vi "Overlay Results (Circle).vi"(5 "Setup":T2, 7 "ROI Descriptor":T1 {"Contours"."Type" items=["No Selection", "Point", "Line", "Rectangle", "Oval", "Polygon", "Free", "Annulus", "Unused2", "Unused3", "Broken Line", "Free Hand Line", "Rotated Rectangle"]}, 8 "Search Lines":T3(array[cluster]) {"?"."Y" format="%.2f"; "?"."X" format="%.2f"; "?"."Y" format="%.2f"; "?"."X" format="%.2f"}, 9 "All Edges Found":cluster{"X":sgl, "Y":sgl}[](array[cluster])=[{"X"=27.450102, "Y"=144.0}, {"X"=70.80146, "Y"=144.0}, {"X"=114.11963, "Y"=144.0}, {"X"=158.60345, "Y"=144.0}, {"X"=202.3678, "Y"=144.0}, {"X"=246.04292, "Y"=144.0}, {"X"=291.42203, "Y"=144.0}, {"X"=336.54822, "Y"=144.0}, {"X"=379.2348, "Y"=144.0}, {"X"=425.02194, "Y"=144.0}, {"X"=467.72144, "Y"=144.0}, {"X"=26.88918, "Y"=210.0}, {"X"=70.6191, "Y"=210.0}, {"X"=115.31038, "Y"=210.0}, {"X"=159.03351, "Y"=210.0}, {"X"=202.2118, "Y"=210.0}, {"X"=247.37573, "Y"=210.0}, {"X"=292.001, "Y"=210.0}, {"X"=336.55954, "Y"=210.0}, {"X"=379.72208, "Y"=210.0}, {"X"=424.86005, "Y"=210.0}, {"X"=468.8485, "Y"=210.0}, {"X"=26.897532, "Y"=309.0}, {"X"=70.88008, "Y"=309.0}, {"X"=114.93419, "Y"=309.0}, {"X"=159.13483, "Y"=309.0}, {"X"=203.12064, "Y"=309.0}, {"X"=247.9202, "Y"=309.0}, {"X"=291.07425, "Y"=309.0}, {"X"=335.25354, "Y"=309.0}, {"X"=378.88284, "Y"=309.0}, {"X"=424.06085, "Y"=309.0}, {"X"=469.80658, "Y"=309.0}] {"Y" format="%.2f"; "X" format="%.2f"}, 10 "Circle":T4 {"Radius" format="%.2f"; "Center"."Y" format="%.2f"; "Center"."X" format="%.2f"}, 11 "Image In":T5) -> (3 "Image Out":T5)   [LabVIEW 2020]
uses:
  IMAQ Image.ctl
panel:
  in  "Result Color":u32(colorbox)=16711680
  in  "Edge Locations Color":u32(colorbox)=16776960
  in  "Search Lines Color":u32(colorbox)=26367
  in  "Search Area Color":u32(colorbox)=65280
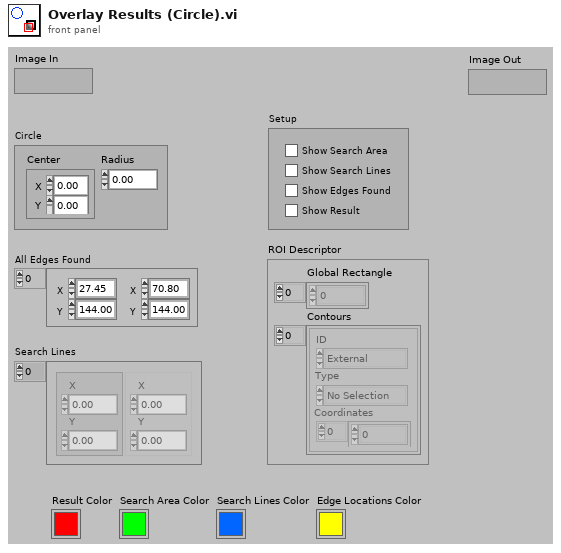
[diagram p1: front panel]
types:
  T1 = cluster{"Global Rectangle":i32[], "Contours":cluster{"ID":enum32{"External", "Internal"}, "Type":u32, "Coordinates":i32[]}[]}
  T2 = cluster{"Show Search Area":bool, "Show Search Lines":bool, "Show Edges Found":bool, "Show Result":bool}
  T3 = cluster{cluster{"X":sgl, "Y":sgl}, cluster{"X":sgl, "Y":sgl}}[]
  T4 = cluster{"Center":cluster{"X":sgl, "Y":sgl}, "Radius":dbl}
  T5 = typedef "IMAQ Image.ctl" = refnum<image>
  T6 = cluster{"[0]":sgl, "[1]":sgl, "[2]":sgl, "[3]":sgl}
  T7 = cluster{"[0]":dbl, "[1]":dbl, "[2]":dbl, "[3]":dbl}
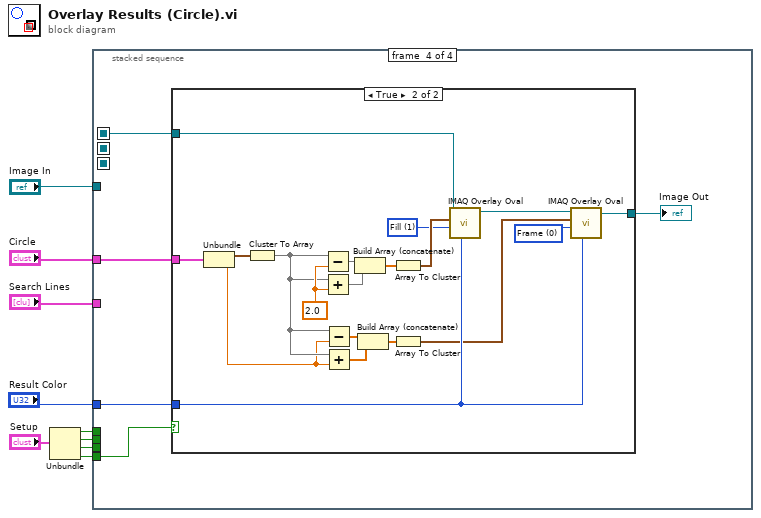
[diagram p0: block diagram]
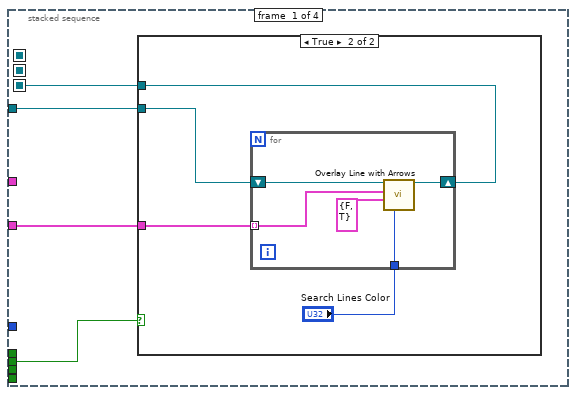
[diagram p2: hidden frame]
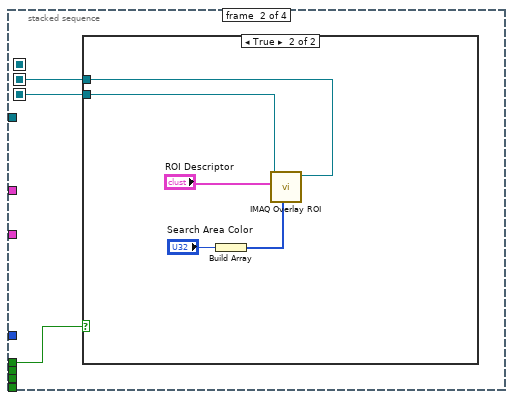
[diagram p4: hidden frame]
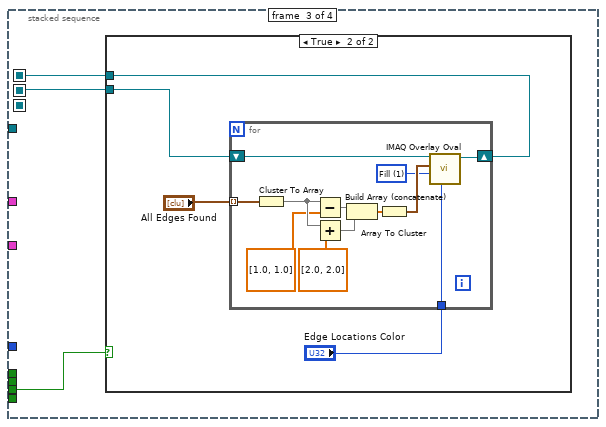
[diagram p6: hidden frame]
diagram:
  n1 = Unbundle("Setup") -> ("Show Search Area"=w3:bool, "Show Search Lines"=w4:bool, "Show Edges Found"=w2:bool, "Show Result"=w1:bool)
  n2 = stacked-sequence {
    seq-local: [_ _ w35 _] -> [_ _ _ w57]
    seq-local: [w12 _ _ _] -> [_ w25 _ _]
    seq-local: [_ w26 _ _] -> [_ _ w34 _]
    tunnel: "Image In" -> [w13 _ _ _]
    tunnel: "Search Lines" -> [w11 _ _ _]
    tunnel: "Result Color" -> [_ _ _ w56]
    tunnel: "Circle" -> [_ _ _ w55]
    tunnel: w4 -> [w10 _ _ _]
    tunnel: w3 -> [_ w24 _ _]
    tunnel: w2 -> [_ _ w33 _]
    tunnel: w1 -> [_ _ _ w54]
    frame #0 {
      n3 = case shown="True" w10 {
        tunnel: w13 -> [w14 w18]
        tunnel: [w14 w16] -> w12
        tunnel: w11 -> [_ w15]
        frame False {
        }
        frame True {
          n4 = for {
            shift-right: [w22] -> w16
            shift-left: w18 -> [w23]
            tunnel: "Search Lines Color" -> [w19]
            tunnel: w15 -> [w21] mode=indexing
            n5 = call "Overlay Line with Arrows.vi"("Color"=w19, "Arrows"=cluster{"Start point":bool, "End point":bool} {"Start point"=FALSE, "End point"=TRUE}, "Line Coordinates"=w21, "Image In"=w23) -> ("Image Out"=w22:T5)  [unwired: 2 in, 5 out]
          }
        }
      }
    }
    frame #1 {
      n6 = case shown="True" w24 {
        tunnel: [w27 w31] -> w26
        tunnel: w25 -> [w27 w32]
        frame False {
        }
        frame True {
          n7 = Build Array("Search Area Color") -> (w28:u32[])
          n8 = call "IMAQ Overlay ROI"("Colors (Green)"=w28, "ROI Descriptor"="ROI Descriptor", "Image"=w32) -> ("Image Out"=w31:T5)  [unwired: 3 in, 5 out]
        }
      }
    }
    frame #2 {
      n9 = case shown="True" w33 {
        tunnel: [w36 w37] -> w35
        tunnel: w34 -> [w36 w38]
        frame False {
        }
        frame True {
          n10 = for {
            shift-right: [w51] -> w37
            shift-left: w38 -> [w52]
            tunnel: "All Edges Found" -> [w50] mode=indexing
            tunnel: "Edge Locations Color" -> [w44]
            w41 = u32 1 items=["Frame", "Fill"] ("Drawing Mode (Frame)")
            n11 = Cluster To Array(cluster=w50) -> (array=w49:sgl[])
            n12 = Subtract(x=w49, y=sgl[] [1.0, 1.0]) -> (x-y=w48:sgl[])
            n13 = Add(x=w49, y=sgl[] [2.0, 2.0]) -> (x+y=w47:sgl[])
            n14 = Build Array (concatenate)(w48, w47) -> (w46:sgl[])
            n15 = Array To Cluster(array=w46) -> (cluster=w45:T6)
            n16 = call "IMAQ Overlay Oval"("Color"=w44, "Drawing Mode (Frame)"=w41, "Bounding Rectangle"=w45, "Image"=w52) -> ("Image Out"=w51:T5)  [unwired: 2 in, 5 out]
          }
        }
      }
    }
    frame #3 {
      n17 = case shown="True" w54 {
        tunnel: w57 -> [w58 w71]
        tunnel: w56 -> [_ w68]
        tunnel: w55 -> [_ w77]
        tunnel: [w58 w69] -> w53
        frame False {
        }
        frame True {
          w59 = u32 0 items=["Frame", "Fill"] ("Drawing Mode (Frame)")
          w60 = u32 1 items=["Frame", "Fill"] ("Drawing Mode (Frame)")
          w67 = sgl 2.0 ("X")
          n18 = Unbundle(w77) -> ("Center"=w72:cluster{"X":sgl, "Y":sgl}, "Radius"=w61:dbl)
          n19 = Cluster To Array(cluster=w72) -> (array=w66:sgl[])
          n20 = Subtract(x=w66, y=w67) -> (x-y=w76:sgl[])
          n21 = Add(x=w66, y=w67) -> (x+y=w75:sgl[])
          n22 = Subtract(x=w66, y=w61) -> (x-y=w64:dbl[])
          n23 = Add(x=w66, y=w61) -> (x+y=w63:dbl[])
          n24 = Build Array (concatenate)(w76, w75) -> (w74:sgl[])
          n25 = Build Array (concatenate)(w64, w63) -> (w65:dbl[])
          n26 = Array To Cluster(array=w74) -> (cluster=w73:T6)
          n27 = Array To Cluster(array=w65) -> (cluster=w62:T7)
          n28 = call "IMAQ Overlay Oval"("Color"=w68, "Drawing Mode (Frame)"=w60, "Bounding Rectangle"=w73, "Image"=w71) -> ("Image Out"=w70:T5)  [unwired: 2 in, 5 out]
          n29 = call "IMAQ Overlay Oval"("Color"=w68, "Drawing Mode (Frame)"=w59, "Bounding Rectangle"=w62, "Image"=w70) -> ("Image Out"=w69:T5)  [unwired: 2 in, 5 out]
        }
      }
      "Image Out" <- w53
    }
  }
